vi "Read acquisition type (Normal).vi"(8 "error in (no error)":errorcluster, 11 "Configure Acquisition Type Msg in":refnum<class "Configure Acquisition Type Msg.lvclass">) -> (0 "error out":errorcluster, 2 "acquisition type (Normal)":i32(ring) items=["Normal", "Peak Detect", "High Resolution", "Envelope", "Average"], 3 "Configure Acquisition Type Msg out":refnum<class "Configure Acquisition Type Msg.lvclass">)   [LabVIEW 2015, in "CS++Scope.lvlib" / "Configure Acquisition Type Msg.lvclass"]
uses:
  Configure Acquisition Type Msg.lvclass
  Configure Acquisition Type Msg.lvclass/Configure Acquisition Type Msg.ctl
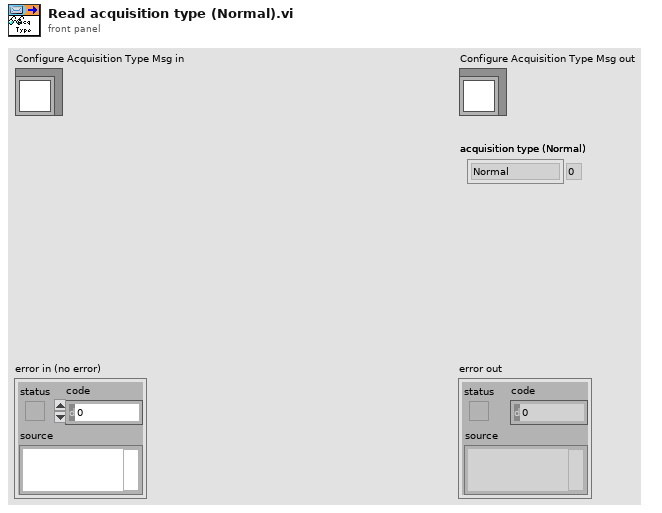
[diagram p1: front panel]
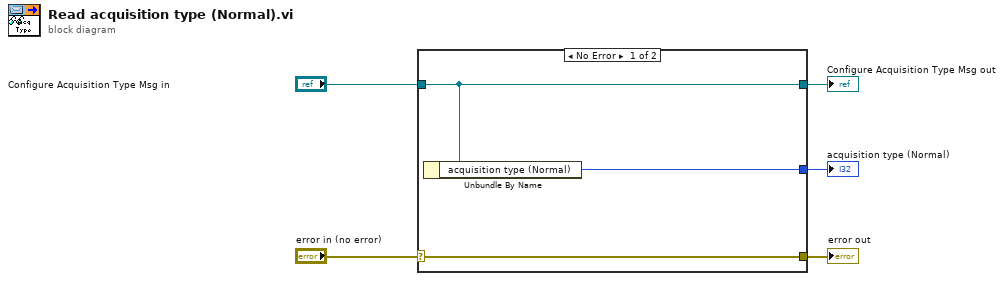
[diagram p0: block diagram]
diagram:
  n1 = case shown="No Error" "error in (no error)" {
    selector: "error in (no error)" -> [w8 w9]
    tunnel: [w8 w9] -> w4
    tunnel: [w7 w10] -> w2
    tunnel: "Configure Acquisition Type Msg in" -> [w7 w10]
    tunnel: [w6 _] -> w1
    frame No Error {
      n2 = Unbundle By Name(w7) -> ("acquisition type (Normal)"=w6:i32)
    }
    frame Error {
    }
  }
  "error out" <- w4
  "Configure Acquisition Type Msg out" <- w2
  "acquisition type (Normal)" <- w1
